vi "oneElectron_chaos_0.0.vi"() -> ()   [LabVIEW 2014]
uses:
  <vilib>/Analysis/baseanly.llb/Mean (DBL).vi
  <vilib>/Analysis/NI_AALBase.lvlib
  common/crest/LabVIEW/LV14/libcommon-crest.lvlib
panel:
  in  "Stiop":bool
  in  "!CHAOS WAN url":string="192.168.150.91:8081"
  out "D2/D1 int":dbl
  out "D2Int":i32
  out "D1Int":i32
  out "sigma main":dbl
  out "mean":dbl format="%0.2f"
  in  "mode":bool
  out "D2":dbl
  out "D1":dbl
  out "Ratio D2/D3":dbl format="%#_4g"
  in  "XY1":bool caption="XY1/XY2"
  in  "Th(streap)":dbl=3.0
  in  "gussConvolution":bool
  in  "Boolean 3":bool
  out "Int # ele":dbl format="%.2e"
  out "dtr":dbl
  out "# ele":dbl format="%0.2f"
  in  "odo/silci":bool=TRUE
  out "s (e-)":dbl format="%_2f"
  out "daq/trigger":bool
  out "RUN (min)":dbl format="%_2g"
  out "m (e-)":dbl format="%_2f"
  in  "fit to [mm]":dbl=48.0 min=0.0 max=48.0 step=3.0
  in  "fit from [mm]":dbl=3.0 min=0.0 max=48.0 step=3.0
  out "X s [mm]":dbl=13.351557326910907 format="%.2f"
  out "X m [mm]":dbl format="%.2f"
  out "XY Graph 4":cluster{cluster{ext, ext}[]}[](graph)=[{[{-1.23749999999999999996, 20683.70651828949}, {1.23749999999999999996, 28639.086891734318}, {3.7124999999999999999, 38314.7910249274}, {6.1875, 49527.93820285375}, {8.6624999999999999995, 61860.08763796215}, {11.1375, 74653.0071654193}, {13.6125, 87048.35655302092}, {16.0875, 98073.19855927354}, {18.5625, 106761.97442709374}, {21.0375, 112294.72297293894}, {23.512499999999999999, 114124.42256243256}, {25.9875, 112066.1190175102}, {28.4625, 106327.73555049808}, {30.9375, 97475.45958787046}, {33.412499999999999999, 86341.68344785097}, {35.8875, 73896.22049364916}, {38.3625, 61108.33274446655}, {40.837499999999999998, 48826.44859679062}, {43.3125, 37695.2243946612}, {45.787499999999999999, 28118.621308150327}]}, {[{0.0, 23638.248164752469393}, {3.0, 27751.287928519853608}, {6.0, 48931.906139470509913}, {9.0, 71021.799624060018857}, {12.0, 85095.41160691138907}, {15.0, 89513.8891360594007}, {18.0, 107920.012194895250786}, {21.0, 119528.82977855355239}, {24.0, 107828.673146201570773}, {27.0, 104829.77465103221442}, {30.0, 102667.51811452324222}, {33.0, 92024.856401616183234}, {36.0, 64831.921624424112338}, {39.0, 48058.523112633217153}, {42.0, 56110.376817814268747}, {45.0, 30116.842769279687985}]}, {[{0.0, 23331.751835247530607}, {3.0, 27419.112071480242435}, {6.0, 48490.493860529382403}, {9.0, 70489.8003759402489}, {12.0, 84512.98839308831407}, {15.0, 88916.510863940302443}, {18.0, 107263.987805104749214}, {21.0, 118838.370221446837604}, {24.0, 107172.926853798784293}, {27.0, 104183.22534896778558}, {30.0, 102027.681885477089565}, {33.0, 91419.143598383496624}, {36.0, 64323.678375575689756}, {39.0, 47621.076887366614045}, {42.0, 55637.623182185731253}, {45.0, 29770.757230720215972}]}]
  in  "Boolean 2":bool
  in  "reset":bool=TRUE
  out "Y s [mm]":dbl=13.351557326910907 format="%.2f"
  out "Y m [mm]":dbl format="%.2f"
  in  "fit to [mm]":dbl=48.0 min=0.0 max=48.0 step=3.0
  in  "fit from [mm]":dbl=3.0 min=0.0 max=48.0 step=3.0
  out "XY Graph 3":cluster{cluster{ext, ext}[]}[](graph)=[{[{-1.23749999999999999996, 20683.70651828949}, {1.23749999999999999996, 28639.086891734318}, {3.7124999999999999999, 38314.7910249274}, {6.1875, 49527.93820285375}, {8.6624999999999999995, 61860.08763796215}, {11.1375, 74653.0071654193}, {13.6125, 87048.35655302092}, {16.0875, 98073.19855927354}, {18.5625, 106761.97442709374}, {21.0375, 112294.72297293894}, {23.512499999999999999, 114124.42256243256}, {25.9875, 112066.1190175102}, {28.4625, 106327.73555049808}, {30.9375, 97475.45958787046}, {33.412499999999999999, 86341.68344785097}, {35.8875, 73896.22049364916}, {38.3625, 61108.33274446655}, {40.837499999999999998, 48826.44859679062}, {43.3125, 37695.2243946612}, {45.787499999999999999, 28118.621308150327}]}, {[{0.0, 23638.248164752469393}, {3.0, 27751.287928519853608}, {6.0, 48931.906139470509913}, {9.0, 71021.799624060018857}, {12.0, 85095.41160691138907}, {15.0, 89513.8891360594007}, {18.0, 107920.012194895250786}, {21.0, 119528.82977855355239}, {24.0, 107828.673146201570773}, {27.0, 104829.77465103221442}, {30.0, 102667.51811452324222}, {33.0, 92024.856401616183234}, {36.0, 64831.921624424112338}, {39.0, 48058.523112633217153}, {42.0, 56110.376817814268747}, {45.0, 30116.842769279687985}]}, {[{0.0, 23331.751835247530607}, {3.0, 27419.112071480242435}, {6.0, 48490.493860529382403}, {9.0, 70489.8003759402489}, {12.0, 84512.98839308831407}, {15.0, 88916.510863940302443}, {18.0, 107263.987805104749214}, {21.0, 118838.370221446837604}, {24.0, 107172.926853798784293}, {27.0, 104183.22534896778558}, {30.0, 102027.681885477089565}, {33.0, 91419.143598383496624}, {36.0, 64323.678375575689756}, {39.0, 47621.076887366614045}, {42.0, 55637.623182185731253}, {45.0, 29770.757230720215972}]}]
  out "#2":i32(slide) scale=0.0..40.0
  out "#1":i32(slide) scale=0.0..40.0
  out "#0":i32(slide)=40 scale=0.0..40.0
  in  "Boolean":bool
  in  "sigle electron":dbl=203.0 format="%3.3f"
  out "ADC Saturation":bool
  out "XY Graph 2":cluster{i32[], i32[]}(graph)
  out "XY Graph":cluster{i32[], dbl[]}(graph)
  in  "ch (calo)":i32=4
  out "Trigger":i32=1696310
  # "Spectra"
  # "horizontal"
  # "vertical"
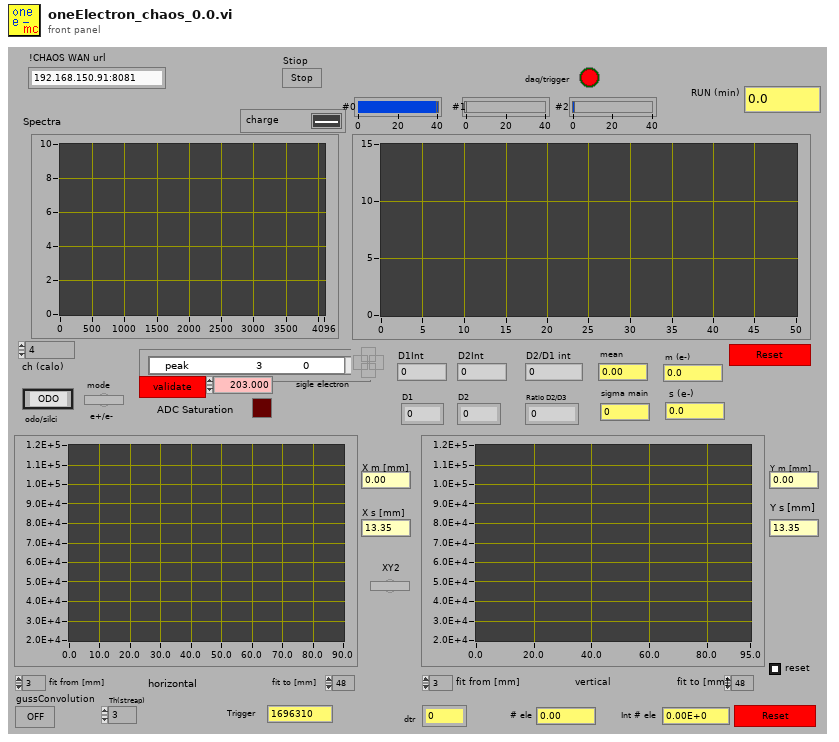
[diagram p1: front panel]
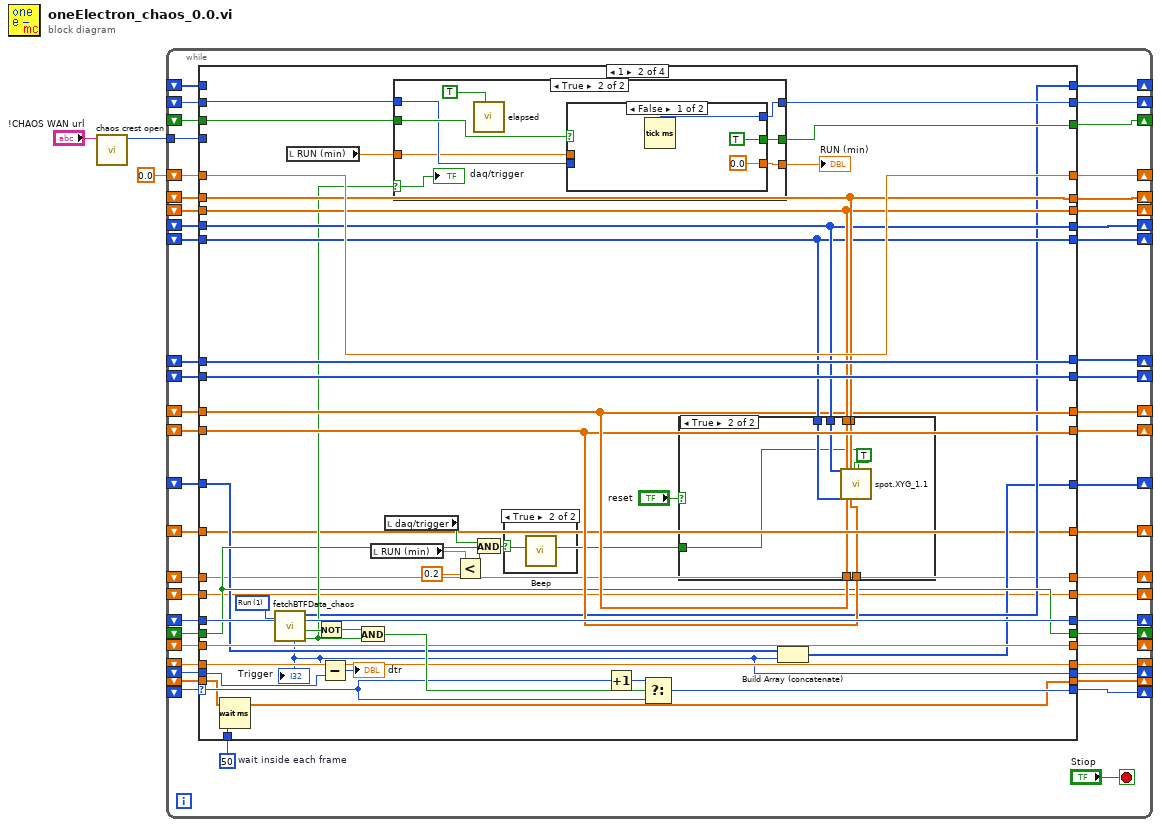
[diagram p0: block diagram]
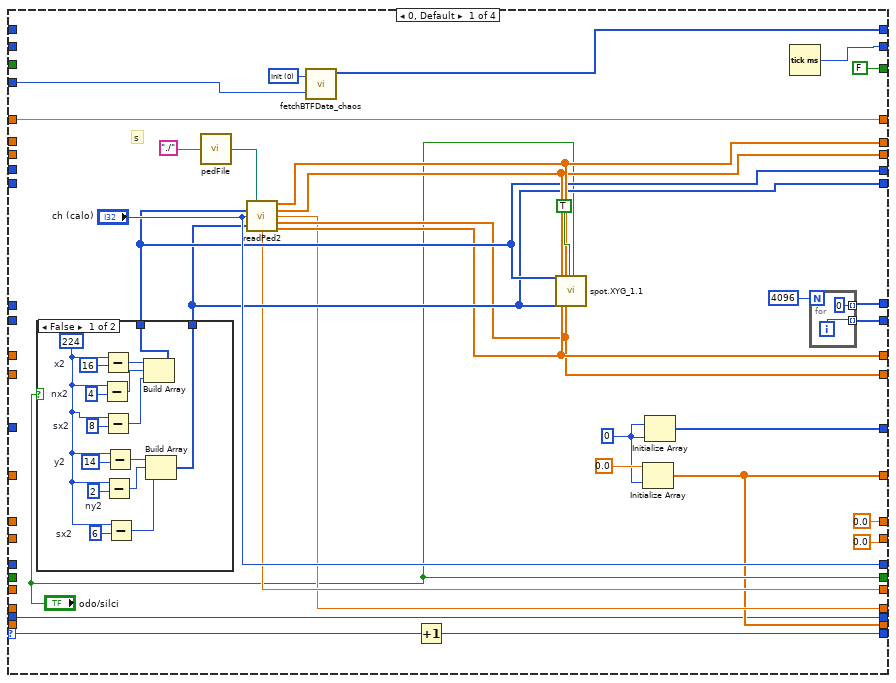
[diagram p2: hidden frame]
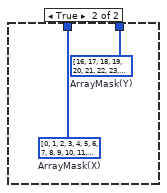
[diagram p3: hidden frame]
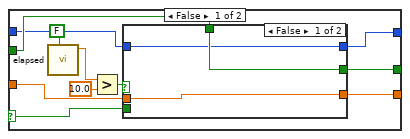
[diagram p5: hidden frame]
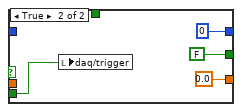
[diagram p6: hidden frame]
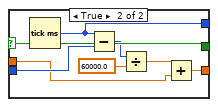
[diagram p7: hidden frame]
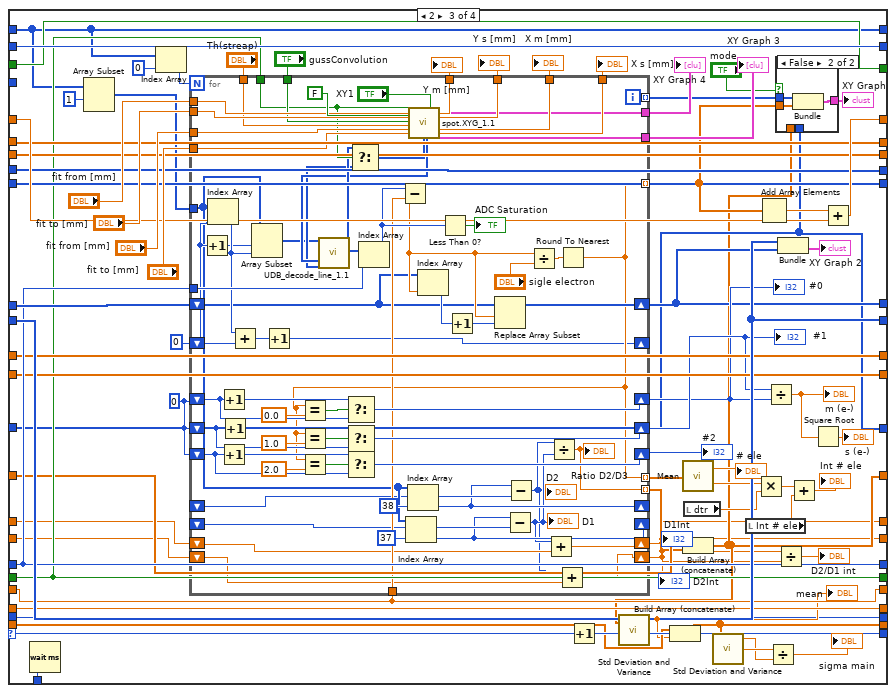
[diagram p9: hidden frame]
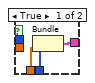
[diagram p10: hidden frame]
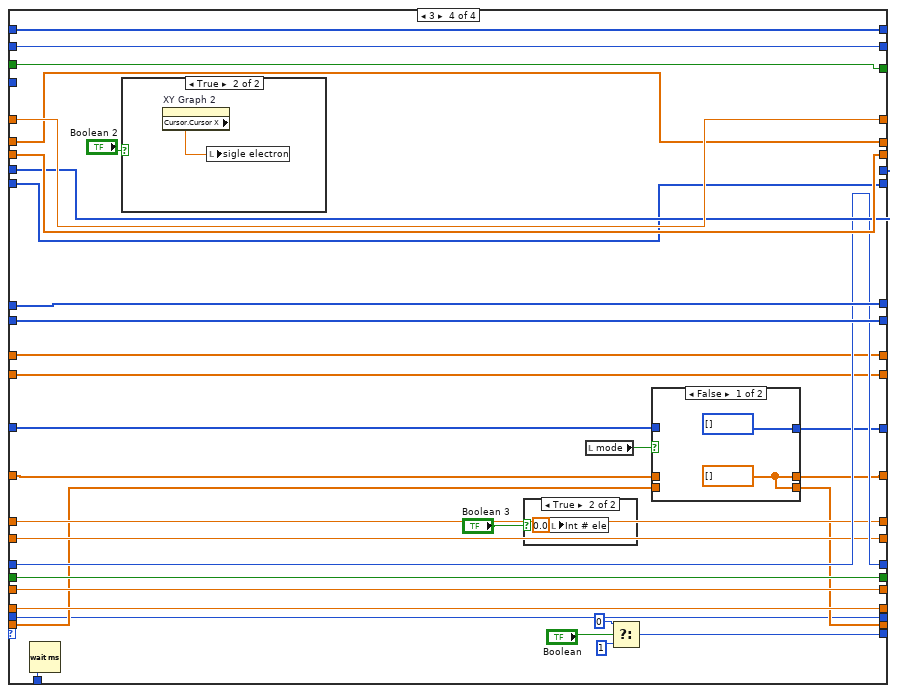
[diagram p11: hidden frame]
diagram:
  n1 = call "chaos crest open.vi"("chaoswanurl"="!CHAOS WAN url") -> ("handleConnection"=w1:u32)  [unwired: 10 in]
  n2 = while {
    shift-left: _ -> [w49]
    shift-right: [w47] -> _
    shift-left: _ -> [w50]
    shift-right: [w48] -> _
    shift-left: _ -> [w51]
    shift-right: [w52] -> _
    shift-left: 0 -> [w13]
    shift-right: [w53] -> _
    shift-right: [w46] -> _
    shift-left: 0.0 -> [w45]
    shift-right: [w44] -> _
    shift-left: _ -> [w43]
    shift-right: [w42] -> _
    shift-left: _ -> [w36]
    shift-right: [w41] -> _
    shift-left: _ -> [w35]
    shift-right: [w40] -> _
    shift-left: _ -> [w34]
    shift-right: [w39] -> _
    shift-left: _ -> [w33]
    shift-right: [w38] -> _
    shift-left: _ -> [w32]
    shift-right: [w37] -> _
    shift-left: _ -> [w31]
    shift-right: [w30] -> _
    shift-left: _ -> [w28]
    shift-right: [w29] -> _
    shift-left: _ -> [w27]
    shift-right: [w26] -> _
    shift-left: _ -> [w25]
    shift-right: [w24] -> _
    shift-left: _ -> [w23]
    shift-right: [w22] -> _
    shift-left: _ -> [w21]
    shift-right: [w20] -> _
    shift-left: _ -> [w17]
    shift-right: [w19] -> _
    shift-left: _ -> [w18]
    shift-right: [w16] -> _
    shift-left: _ -> [w15]
    shift-right: [w10] -> _
    shift-left: _ -> [w12]
    shift-right: [w9] -> _
    shift-left: _ -> [w11]
    shift-right: [w8] -> _
    shift-left: _ -> [w7]
    tunnel: w1 -> [w6]
    stop <- "Stiop" stop-if-true
    w14 = u32 50  # wait inside each frame
    n3 = case shown="1" w13 {
      selector: w13 -> [w84 w142 w254 _]
      tunnel: [w81 w144 w253 w368] -> w53
      tunnel: [w61 w113 w215 w365] -> w52
      tunnel: w51 -> [_ _ w215 w365]
      tunnel: w43 -> [_ w132 w240 w358]
      tunnel: w50 -> [_ w140 w263 w367]
      tunnel: w49 -> [_ w139 w262 w366]
      tunnel: [w83 w140 w227 w367] -> w48
      tunnel: [w82 w139 w262 w366] -> w47
      tunnel: [w79 w137 w246 w363] -> w46
      tunnel: w45 -> [w79 w137 w245 w363]
      tunnel: ["ch (calo)" w132 w240 w358] -> w44
      tunnel: [w75 w136 w244 w362] -> w42
      tunnel: [w74 w135 w243 w361] -> w41
      tunnel: [w73 w134 w242 w360] -> w40
      tunnel: [w72 w133 w241 w359] -> w39
      tunnel: [w71 w131 w239 w357] -> w38
      tunnel: [w70 w130 w238 w356] -> w37
      tunnel: w36 -> [_ w136 w244 w362]
      tunnel: w35 -> [_ w135 w243 w361]
      tunnel: w34 -> [_ w134 w242 w360]
      tunnel: w33 -> [_ w133 w241 w359]
      tunnel: w32 -> [_ w131 w239 w357]
      tunnel: w31 -> [_ w130 w238 w356]
      tunnel: [w69 w129 w236 w355] -> w30
      tunnel: [w68 w128 w237 w354] -> w29
      tunnel: w28 -> [_ w129 w236 w355]
      tunnel: w27 -> [_ w128 w237 w354]
      tunnel: [w67 w125 w235 w353] -> w26
      tunnel: w25 -> [_ w124 w235 w353]
      tunnel: [FALSE w122 w234 w352] -> w24
      tunnel: w23 -> [_ w123 w234 w352]
      tunnel: ["odo/silci" w115 w228 w351] -> w22
      tunnel: w21 -> [_ w115 w228 w351]
      tunnel: [w60 w110 w204 w344] -> w20
      tunnel: [w62 w111 w207 w343] -> w19
      tunnel: w18 -> [_ w112 w207 w342]
      tunnel: w17 -> [_ w110 w212 w341]
      tunnel: [w60 w109 w203 w345] -> w16
      tunnel: w15 -> [_ w109 w206 w340]
      tunnel: w14 -> [_ w108 w199 w349]
      tunnel: w12 -> [_ w107 w197 w348]
      tunnel: w11 -> [_ w106 w196 w347]
      tunnel: [0.0 w107 w195 w348] -> w10
      tunnel: [0.0 w106 w194 w347] -> w9
      tunnel: [w55 w105 w193 w339] -> w8
      tunnel: w7 -> [w55 w104 w193 w339]
      tunnel: w6 -> [w54 _ _ _]
      frame 0, Default {
        w56 = 0 ("index")
        w64 = u16 0 items=["Init", "Run"] ("Funcion")
        # "s"
        n4 = case shown="False" "odo/silci" {
          tunnel: [w95 w101] -> w73
          tunnel: [w90 w100] -> w72
          frame False {
            w87 = 6  # sx2
            w89 = 8  # sx2
            w92 = 2  # ny2
            w93 = 14  # y2
            w98 = 4  # nx2
            w97 = 16  # x2
            w86 = 224 ("element")
            n5 = Subtract(x=w86, y=w98) -> (x-y=w99:i32)
            n6 = Subtract(x=w86, y=w97) -> (x-y=w96:i32)
            n7 = Subtract(x=w86, y=w89) -> (x-y=w88:i32)
            n8 = Subtract(x=w86, y=w92) -> (x-y=w91:i32)
            n9 = Subtract(x=w86, y=w93) -> (x-y=w94:i32)
            n10 = Subtract(x=w86, y=w87) -> (x-y=w85:i32)
            n11 = Build Array(w96, w99, w88) -> (w95:i32[])
            n12 = Build Array(w94, w91, w85) -> (w90:i32[])
          }
          frame True {
            w101 = i32[] [0, 1, 2, 3, 4, 5, 6, 7, 8, 9, 10, 11, 12, 13, 14, 15]  # ArrayMask(X)
            w100 = i32[] [16, 17, 18, 19, 20, 21, 22, 23, 24, 25, 26, 27, 28, 29, 30, 31]  # ArrayMask(Y)
          }
        }
        n13 = call "pedFile.vi"("pattern"="./") -> ("last Ped File"=w77:path)  [unwired: 4 in]
        n14 = call "readPed2.vi"("file path (dialog if empty)"=w77, "mask 1"=w73, "calo ch"="ch (calo)", "mask 2"=w72) -> ("ped 1"=w75:sgl[], "sigma 1"=w74:sgl[], "vcm ped"=w68:sgl, "ped 2"=w70:sgl[], "caloped"=w69:sgl, "sigma 2"=w71:sgl[])  [unwired: 5 in, 1 out]
        n15 = call "fetchBTFData_chaos.vi"("Funcion"=w64, "!CHAOS WAN url"=w54) -> ("Array"=w61:i32[])  [unwired: 2 in, 3 out]
        n16 = Increment(x=w84) -> (x+1=w81:i32)
        n17 = call "spot.XYG_1.1.vi"("ArrayMask(X)"=w73, "ArrayMask(Y )"=w72, "sigmaPed(x)"=w74, "sigmaPed(Y)"=w71, "Ped(x)"=w75, "Ped(Y)"=w70, "init?"=TRUE, "odo/sili"="odo/silci") -> ()  [unwired: 14 in, 6 out]
        n18 = Initialize Array(0.0 ("index"), w56) -> (w60:dbl[])
        n19 = Initialize Array(w56, w56) -> (w62:i32[])
        n20 = Tick Count (ms)() -> (millisecond timer value=w67:u32)
        n21 = for {
          N: 4096 -> [_]
          tunnel: [w103] -> w82 mode=indexing
          tunnel: [0] -> w83 mode=indexing
          i -> [w103]
        }
      }
      frame 1 {
        w147 = u16 1 items=["Init", "Run"] ("Funcion")
        n22 = Wait (ms)(milliseconds to wait=w108) -> ()  [unwired: 1 out]
        n23 = call "fetchBTFData_chaos.vi"("Funcion"=w147) -> ("lastTrigger"=w105:i32, "Array"=w113:i32[], "ReadError"=w146:bool, "DataReady"=w116:bool)  [unwired: 3 in]
        "Trigger" <- w105
        n24 = local read "RUN (min)"() -> (w126:dbl)
        n25 = Not(x=w146) -> (.not. x?=w145:bool)
        n26 = Subtract(x=w105, y=w104) -> (x-y=→"dtr":i32)
        n27 = And(x=w145, y=w116) -> (x .and. y?=w143:bool)
        n28 = local read "RUN (min)"() -> (w120:dbl)
        n29 = local read "daq/trigger"() -> (w118:bool)
        n30 = case shown="True" w116 {
          selector: w116 -> [w154 w166]
          tunnel: [w153 w171] -> w127
          tunnel: w126 -> [w152 w167]
          tunnel: [w149 w172] -> w125
          tunnel: w124 -> [w148 w168]
          tunnel: w123 -> [w150 w173]
          tunnel: [w151 w169] -> w122
          frame False {
            n31 = call "elapsed.vi"("INIT?"=FALSE) -> ("sec"=w157:dbl)  [unwired: 6 in, 1 out]
            n32 = Greater?(x=w157, y=10.0) -> (0:w155:bool)
            n33 = case shown="False" w155 {
              tunnel: w154 -> [_ w165]
              tunnel: [w161 0.0] -> w153
              tunnel: w152 -> [w161 _]
              tunnel: [w160 FALSE] -> w151
              tunnel: w150 -> [w160 _]
              tunnel: [w159 u32 0 ("millisecond timer value")] -> w149
              tunnel: w148 -> [w159 _]
              frame False {
              }
              frame True {
                n34 = local write "daq/trigger"(w165) -> ()
              }
            }
          }
          frame True {
            n35 = call "elapsed.vi"("INIT?"=TRUE) -> ()  [unwired: 6 in, 2 out]
            n36 = case shown="False" w173 {
              selector: w173 -> [_ w184]
              tunnel: [w176 w177] -> w172
              tunnel: [0.0 w181] -> w171
              tunnel: [TRUE w184] -> w169
              tunnel: w168 -> [_ w183]
              tunnel: w167 -> [_ w180]
              frame False {
                n37 = Tick Count (ms)() -> (millisecond timer value=w176:u32)
              }
              frame True {
                n38 = Tick Count (ms)() -> (millisecond timer value=w177:u32)
                n39 = Subtract(x=w177, y=w183) -> (x-y=w182:u32)
                n40 = Divide(x=w182, y=60000.0) -> (x/y=w179:dbl)
                n41 = Add(x=w179, y=w180) -> (x+y=w181:dbl)
              }
            }
            "daq/trigger" <- w166
          }
        }
        "RUN (min)" <- w127
        n42 = Less?(x=w120, y=0.2) -> (x < y?=w117:bool)
        n43 = And(x=w118, y=w117) -> (x .and. y?=w119:bool)
        n44 = case shown="True" w119 {
          frame False {
          }
          frame True {
            n45 = call <vilib>:"Beep.vi"() -> ()  [unwired: 12 in]
          }
        }
        n46 = Increment(x=w142) -> (x+1=w141:i32)
        n47 = Select(t=w141, s=w143, f=w142) -> (s? t:f=w144:i32)
        n48 = case shown="True" "reset" {
          tunnel: w136 -> [_ w191]
          tunnel: w135 -> [_ w190]
          tunnel: w134 -> [_ w187]
          tunnel: w133 -> [_ w186]
          tunnel: w131 -> [_ w189]
          tunnel: w130 -> [_ w188]
          tunnel: w115 -> [_ w185]
          frame False {
          }
          frame True {
            n49 = call "spot.XYG_1.1.vi"("ArrayMask(X)"=w187, "ArrayMask(Y )"=w186, "sigmaPed(x)"=w190, "sigmaPed(Y)"=w189, "Ped(x)"=w191, "Ped(Y)"=w188, "init?"=TRUE, "odo/sili"=w185) -> ()  [unwired: 14 in, 6 out]
          }
        }
        n50 = Build Array (concatenate)(w112, w105) -> (w111:i32[])
      }
      frame 2 {
        w261 = 0
        n51 = Wait (ms)(milliseconds to wait=w199) -> ()  [unwired: 1 out]
        n52 = Array Subset(array=w215, index=1) -> (w214:i32[])  [unwired: 1 in]
        n53 = Index Array(array=w215, index=0) -> (element=w216:i32)
        n54 = for {
          N: w216 -> [_]
          tunnel: w214 -> [w283]
          tunnel: [w301] -> w233 mode=indexing
          tunnel: [w338] -> w208 mode=indexing
          tunnel: w240 -> [w337]
          shift-right: [w333] -> w227
          shift-left: w263 -> [w285]
          shift-right: [w319] -> w231
          shift-left: w261 -> [w320]
          shift-right: [w318] -> w232
          shift-left: w261 -> [w321]
          shift-right: [w317] -> w260
          shift-left: w261 -> [w322]
          tunnel: [w307] -> w259
          tunnel: "fit from [mm]" -> [w313]
          tunnel: "fit to [mm]" -> [w312]
          tunnel: [w316] -> w256
          tunnel: [w315] -> w255
          tunnel: [w311] -> w252
          tunnel: [w310] -> w251
          tunnel: "fit from [mm]" -> [w309]
          tunnel: "fit to [mm]" -> [w308]
          tunnel: [w306] -> w248
          tunnel: w236 -> [w304]
          tunnel: w228 -> [w297]
          tunnel: [w301] -> w226 mode=indexing
          tunnel: "gussConvolution" -> [w300]
          tunnel: "Th(streap)" -> [w299]
          shift-right: [w286] -> _
          shift-left: 0 ("index") -> [w287]
          shift-right: [w275] -> _
          shift-left: _ -> [w281]
          shift-right: [w278] -> _
          shift-left: _ -> [w280]
          tunnel: [w279] -> w211 mode=indexing
          shift-right: [w276] -> w195
          shift-left: w197 -> [w277]
          shift-right: [w273] -> w194
          shift-left: w196 -> [w274]
          i -> [w338]
          n55 = Increment(x=w287) -> (x+1=w289:i32)
          n56 = Index Array(array=w283, index=w287) -> (element=w291:i32)
          n57 = Increment(x=w320) -> (x+1=w325:i32)
          n58 = Increment(x=w322) -> (x+1=w323:i32)
          n59 = Increment(x=w321) -> (x+1=w324:i32)
          n60 = Add(x=w291, y=w287) -> (x+y=w290:i32)
          n61 = Array Subset(array=w283, index=w289, length=w291) -> (w288:i32[])
          n62 = Increment(x=w290) -> (x+1=w286:i32)
          n63 = call "UDB_decode_line_1.1.vi"("arrayIn"=w288) -> ("streap"=w294:i32[], "value"=w293:i32[], "qdc1(prof)"=w296:i32[], "qdc2(calo)"=w298:i32[])  [unwired: 3 in, 12 out]
          n64 = Select(t=w296, s=w297, f=w293) -> (s? t:f=w295:i32[])
          n65 = Index Array(array=w298, index=w337) -> (element=w305:i32)
          n66 = Subtract(x=w305, y=w304) -> (x-y=w303:sgl)
          n67 = Index Array(array=w283, index=37) -> (element=w278:i32)
          n68 = Index Array(array=w283, index=38) -> (element=w275:i32)
          n69 = call "spot.XYG_1.1.vi"("fromX"=w313, "toX"=w312, "gussConvolution"=w300, "Th(streap)"=w299, "fromY"=w309, "toY"=w308, "init?"=FALSE, "dataRaw"=w295, "odo/sili"=w297, "STREAP"=w294, "1/2"="XY1") -> ("Y plot"=w306:cluster{cluster{ext, ext}[]}[], "mean Y"=w316:dbl, "sigma Y"=w315:dbl, "mean X"=w311:dbl, "sigmaX"=w310:dbl, "X plot"=w307:cluster{cluster{ext, ext}[]}[])  [unwired: 11 in]
          n70 = Index Array(array=w285, index=w303) -> (element=w335:i32)
          n71 = Less Than 0?(x=w305) -> (x < 0?=→"ADC Saturation":bool)
          n72 = Increment(x=w335) -> (x+1=w336:i32)
          n73 = Replace Array Subset(array=w285, new element=w336, index=w303) -> (w333:i32[])
          n74 = Subtract(x=w278, y=w280) -> (x-y=w272:i32)
          "D1" <- w272
          n75 = Subtract(x=w275, y=w281) -> (x-y=w271:i32)
          "D2" <- w271
          n76 = Divide(x=w303, y="sigle electron") -> (x/y=w332:dbl)
          n77 = Add(x=w272, y=w277) -> (x+y=w276:dbl)
          n78 = Divide(x=w271, y=w272) -> (x/y=w279:dbl)
          "Ratio D2/D3" <- w279
          n79 = Add(x=w271, y=w274) -> (x+y=w273:dbl)
          n80 = Round To Nearest(number=w332) -> (nearest integer value=w301:dbl)
          n81 = Equal?(x=w301, y=0.0) -> (x = y?=w328:bool)
          n82 = Equal?(x=w301, y=1.0) -> (x = y?=w327:bool)
          n83 = Equal?(x=w301, y=2.0) -> (x = y?=w326:bool)
          n84 = Select(t=w325, s=w328, f=w320) -> (s? t:f=w319:i32)
          n85 = Select(t=w324, s=w327, f=w321) -> (s? t:f=w318:i32)
          n86 = Select(t=w323, s=w326, f=w322) -> (s? t:f=w317:i32)
        }
        "#0" <- w231
        "#1" <- w232
        "#2" <- w260
        "XY Graph 3" <- w259
        "Y s [mm]" <- w255
        "Y m [mm]" <- w256
        "XY Graph 4" <- w248
        "X m [mm]" <- w252
        "X s [mm]" <- w251
        "D1Int" <- w195
        "D2Int" <- w194
        n87 = Increment(x=w254) -> (x+1=w253:i32)
        n88 = call-poly <vilib>:"Mean.vi"("X"=w226) -> ("mean"=w225:dbl)  [unwired: 1 out]
        "# ele" <- w225
        n89 = Build Array (concatenate)(w212, w211) -> (w204:dbl[])
        n90 = call <vilib>:"Std Deviation and Variance.vi"("X"=w204) -> ("mean"=w205:dbl)  [unwired: 1 in, 2 out]
        "mean" <- w205
        n91 = Build Array (concatenate)(w206, w205) -> (w203:dbl[])
        n92 = local read "dtr"() -> (w224:dbl)
        n93 = call <vilib>:"Std Deviation and Variance.vi"("X"=w203) -> ("mean"=w201:dbl, "standard deviation"=w202:dbl)  [unwired: 1 in, 1 out]
        n94 = local read "Int # ele"() -> (w221:dbl)
        n95 = Multiply(x=w225, y=w224) -> (x*y=w223:dbl)
        n96 = Add Array Elements(numeric array=w233) -> (sum=w247:dbl)
        n97 = Divide(x=w232, y=w231) -> (x/y=w229:dbl)
        "m (e-)" <- w229
        n98 = Divide(x=w202, y=w201) -> (x/y=→"sigma main":dbl)
        n99 = case shown="False" "mode" {
          tunnel: w233 -> [_ w270]
          tunnel: w208 -> [_ w269]
          tunnel: [w267 w268] -> w210
          tunnel: w207 -> [w266 _]
          tunnel: w204 -> [w265 _]
          frame True {
            n100 = Bundle(w266, w265) -> (w267:cluster{i32[], dbl[]})  [unwired: 1 in]
          }
          frame False {
            n101 = Bundle(w269, w270) -> (w268:cluster{i32[], dbl[]})  [unwired: 1 in]
          }
        }
        "XY Graph" <- w210
        n102 = Divide(x=w194, y=w195) -> (x/y=→"D2/D1 int":dbl)
        n103 = Bundle(w262, w227) -> (→"XY Graph 2":cluster{i32[], i32[]})  [unwired: 1 in]
        n104 = Add(x=w223, y=w221) -> (x+y=→"Int # ele":dbl)
        n105 = Square Root(x=w229) -> (sqrt(x)=→"s (e-)":dbl)
        n106 = Add(x=w247, y=w245) -> (x+y=w246:dbl)
      }
      frame 3 {
        n107 = Wait (ms)(milliseconds to wait=w349) -> ()  [unwired: 1 out]
        n108 = case shown="True" "Boolean 2" {
          frame False {
          }
          frame True {
            n109 = property on="XY Graph 2" class="XYGraph (strict)"() -> ("Cursor.Cursor X"=w378:dbl)  [unwired: 2 in, 2 out]
            n110 = local write "sigle electron"(w378) -> ()
          }
        }
        n111 = case shown="True" "Boolean 3" {
          frame False {
          }
          frame True {
            n112 = local write "Int # ele"(0.0 ("Int # ele")) -> ()
          }
        }
        n113 = local read "mode"() -> (w346:bool)
        n114 = Select(t=0, s="Boolean", f=1) -> (s? t:f=w368:i32)
        n115 = case shown="False" w346 {
          tunnel: [w373 w374] -> w345
          tunnel: [w373 w375] -> w344
          tunnel: [i32[] [] w376] -> w343
          tunnel: w342 -> [_ w376]
          tunnel: w341 -> [_ w375]
          tunnel: w340 -> [_ w374]
          frame False {
            w373 = dbl[] []
          }
          frame True {
          }
        }
      }
    }
  }
